vi "Read from Cluster Ref.vi"(8 "Error In":errorcluster, 10 "array":string[](array[string]), 11 "Cluster Ref In":refnum<vi>) -> (0 "Error Out":errorcluster, 1 "Class Name":string[](array[string]), 2 "Class ID":u32[](array[numeric]), 3 "Value":string[](array[string]), 4 "Label Name":string[](array[string]))   [LabVIEW 2014]
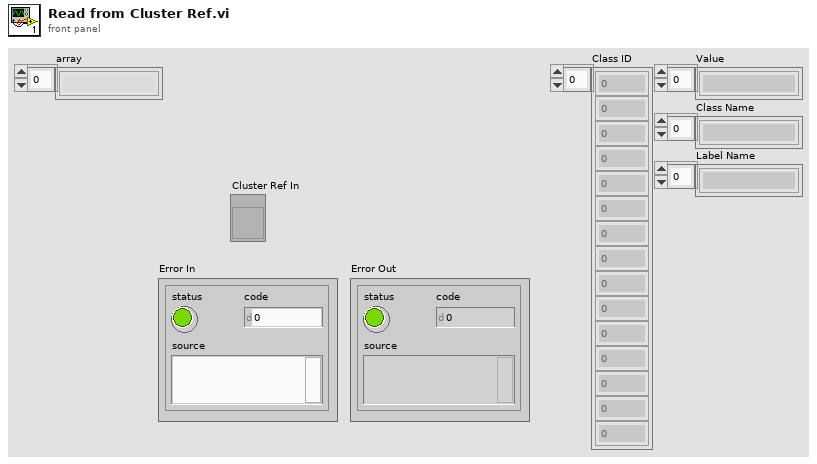
[diagram p1: front panel]
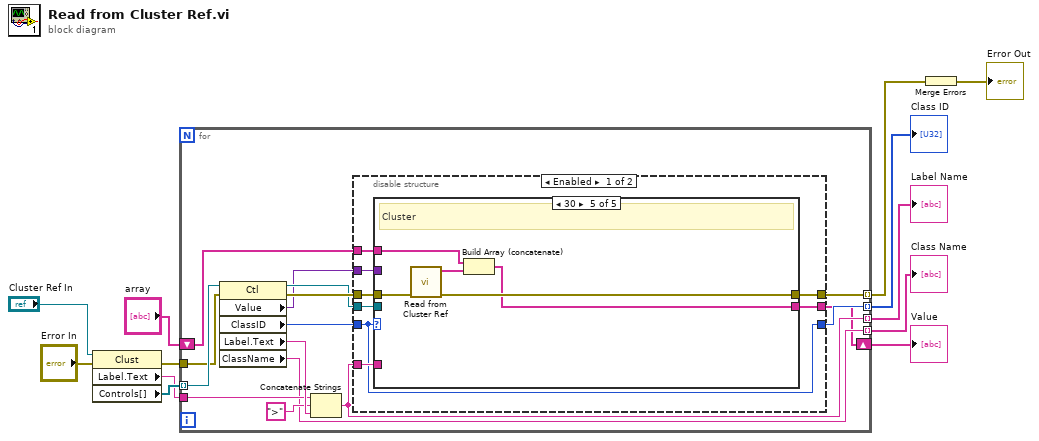
[diagram p0: block diagram]
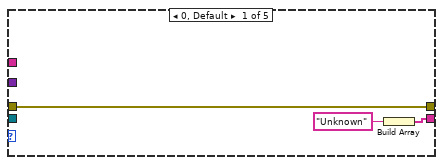
[diagram p2: hidden frame]
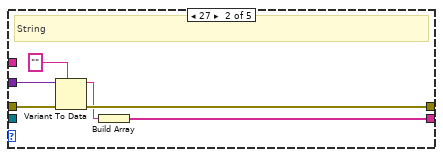
[diagram p3: hidden frame]
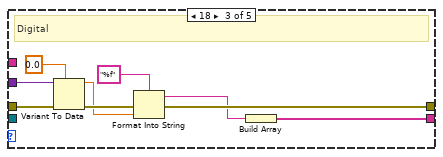
[diagram p4: hidden frame]
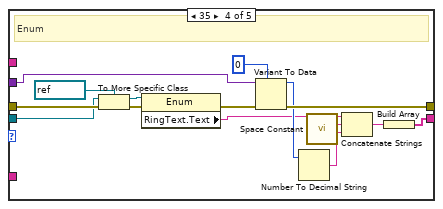
[diagram p5: hidden frame]
diagram:
  n1 = property on="Property Node" class="Clust"(reference="Cluster Ref In", error in="Error In") -> (error out=w8:errorcluster, "Label.Text"=w9:string, "Controls[]"=w12:refnum<vi>[])  [unwired: 1 out]
  n2 = for {
    tunnel: w12 -> [w27] mode=indexing
    tunnel: [w18] -> w11 mode=indexing
    tunnel: w9 -> [w24]
    tunnel: w8 -> [w23]
    tunnel: [w17] -> w7 mode=indexing
    tunnel: [w16] -> w6 mode=indexing
    tunnel: [w15] -> w4 mode=indexing
    shift-right: [w13] -> w1
    shift-left: "array" -> [w14]
    n3 = property class="Ctl"(reference=w27, error in=w23) -> (reference out=w20:refnum<vi>, error out=w21:errorcluster, "Value"=w19:variant, "ClassID"=w22:u32, "Label.Text"=w26:string, "ClassName"=w17:string)
    n4 = Concatenate Strings(w24, ">" ("string"), w26) -> (w16:string)
    n5 = disable-structure shown="Enabled" {
      disable-tunnel: w22 -> [w31 w75]
      disable-tunnel: w21 -> [w35 _]
      disable-tunnel: w20 -> [w34 _]
      disable-tunnel: w16 -> [w33 w74]
      disable-tunnel: w19 -> [w32 _]
      disable-tunnel: [w31 w75] -> w18
      disable-tunnel: [w30 _] -> w15
      disable-tunnel: w14 -> [w29 _]
      disable-tunnel: [w28 _] -> w13
      frame Enabled {
        n6 = case shown="30" w31 {
          tunnel: w35 -> [w38 w44 w53 w68 w73]
          tunnel: w34 -> [_ _ _ w60 _]
          tunnel: w33 -> [_ _ _ _ _]
          tunnel: w32 -> [_ w43 w52 w67 _]
          tunnel: [w38 w41 w49 w65 w72] -> w30
          tunnel: w29 -> [_ _ _ _ w71]
          tunnel: [w36 w40 w46 w55 w69] -> w28
          frame 0, Default {
            n7 = Build Array("Unknown") -> (w36:string[])
          }
          frame 27 {
            # "String"
            n8 = Variant To Data(error in=w44, type="", Variant=w43) -> (data=w39:string, error out=w41:errorcluster)
            n9 = Build Array(w39) -> (w40:string[])
          }
          frame 18 {
            # "Digital"
            n10 = Variant To Data(error in=w53, type=0.0, Variant=w52) -> (data=w48:dbl, error out=w51:errorcluster)
            n11 = Format Into String(format string="%f", error in=w51, w48) -> (resulting string=w45:string, error out=w49:errorcluster)  [unwired: 1 in]
            n12 = Build Array(w45) -> (w46:string[])
          }
          frame 35 {
            # "Enum"
            n13 = To More Specific Class(target class=refnum<vi> refnum ("Enum"), reference=w60, error in=w68) -> (specific class reference=w58:refnum<vi>, error out=w61:errorcluster)
            n14 = property class="Enum"(reference=w58, error in=w61) -> (error out=w62:errorcluster, "RingText.Text"=w57:string)  [unwired: 1 out]
            n15 = Variant To Data(error in=w62, type=i16 0 ("16bit integer"), Variant=w67) -> (data=w64:i16, error out=w65:errorcluster)
            n16 = Number To Decimal String(number=w64) -> (decimal integer string=w63:string)  [unwired: 1 in]
            n17 = call <vilib>:"Space Constant.vi"() -> ("String"=w56:string)
            n18 = Concatenate Strings(w57, w56, w63) -> (w54:string)
            n19 = Build Array(w54) -> (w55:string[])
          }
          frame 30 {
            # "Cluster"
            n20 = call "Read from Cluster Ref.vi"("Error In"=w73) -> ("Error Out"=w72:errorcluster, "Value"=w70:string[])  [unwired: 6 in, 3 out]
            n21 = Build Array (concatenate)(w71, w70) -> (w69:string[])
          }
        }
      }
      frame Disabled {
      }
    }
  }
  "Class ID" <- w11
  "Value" <- w1
  "Class Name" <- w7
  "Label Name" <- w6
  n22 = Merge Errors(w4) -> (→"Error Out":errorcluster)
